vi "calc_params.vi"(5 "Field":dbl, 6 "Dose":dbl, 7 "Frequency":dbl) -> (0 "Optimal negative freq":dbl, 1 "Optimal positive freq":dbl, 2 "K value (rate)":dbl, 3 "Steady state":dbl)   [LabVIEW 2015]
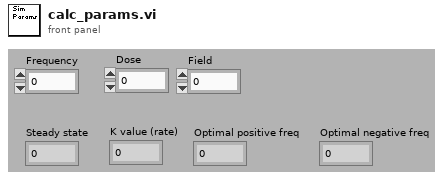
[diagram p1: front panel]
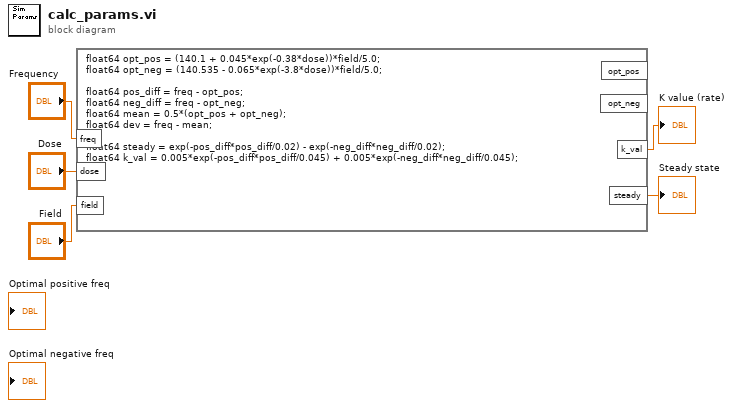
[diagram p0: block diagram]
diagram:
  n1 = formula code="float64 opt_pos = (140.1 + 0.045*exp(-0.38*dose))*field/5.0;\nfloat64 opt_neg = (140.535 - 0.065*exp(-3.8*dose))*field/5.0;\n\nfloat64 pos_diff = freq - opt_pos;\nfloat64 neg_diff = freq - opt_neg;\nfloat64 mean = 0.5*(opt_pos + opt_neg);\nfloat64 dev = freq - mean;\n\nfloat64 steady = exp(-pos_diff*pos_diff/0.02) - exp(-neg_diff*neg_diff/0.02);\nfloat64 k_val = 0.005*exp(-pos_diff*pos_diff/0.045) + 0.005*exp(-neg_diff*neg_diff/0.045);"("freq"="Frequency", "field"="Field", "dose"="Dose") -> ("steady"=→"Steady state":dbl, "k_val"=→"K value (rate)":dbl)  [unwired: 2 out]
